vi "AutoDropStack.vi"() -> (0 "Done?":bool)   [LabVIEW 2014]
uses:
  Elevator/Elevator Control Command.ctl
  Elevator/Elevator Command.ctl
  Common Code/Elevator Mode.ctl
  Robot Global Data.vi
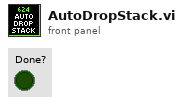
[diagram p1: front panel]
types:
  T1 = typedef "Elevator Command.ctl" = enum16{"Idle", "Load 1", "Load 2", "Load 3", "Drop Stack", "Eject Stack", "Load Trashcan"}
  T2 = typedef "Elevator Mode.ctl" = enum16{"Manual", "Safe", "Auto"}
  T3 = typedef "Elevator Control Command.ctl" = cluster{"Command":T1, "Manual Motor Out":dbl, "Manual Eject Piston":bool, "Mode":T2, "Override Limits":bool, "Manual Stabilizer":bool, "Manual Finger":bool, "Load from Step?":bool, "Store Trashcan?":bool}
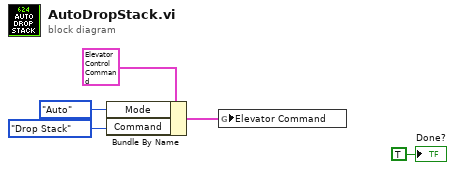
[diagram p0: block diagram]
diagram:
  n1 = Bundle By Name(cluster=T3 {"Command"=enum."Idle", "Manual Motor Out"=0.0, "Manual Eject Piston"=FALSE, "Mode"=enum."Manual", "Override Limits"=FALSE, "Manual Stabilizer"=FALSE, "Manual Finger"=FALSE, "Load from Step?"=FALSE, "Store Trashcan?"=FALSE} ("Elevator Command"), "Mode"=Elevator_Mode."Auto", "Command"=Elevator_Command."Drop Stack") -> (w2:T3)
  n2 = global write "Robot Global Data.vi" "Elevator Command"(w2) -> ()
  "Done?" <- TRUE ("Done?")
